vi "Control Bank Relays.vi"(8 "error in (no error)":errorcluster, 10 "bank params":T1, 11 "Refnum in":T4) -> (0 "error out":errorcluster)   [LabVIEW 2017, in "NI 272x Resistive Simulation Custom Device Engine.lvlib"]
uses:
  NI 272x Resistive Simulation Custom Device Engine.lvlib
  <instrlib>/ni272xReferenceVIs/ni272xReferenceVIs.llb/ni272x Reference.ctl
  bank params.ctl
  <vilib>/NI/NIVS Inline Async API/_Data Access Engine/Data Access Engine/Types/Read.DVR.ctl
  <vilib>/NI/NIVS Inline Async API/_Data Access Engine/Access Type Classes/Read/Read.lvclass
  Controls/Compiled Connect Channel.ctl
  <vilib>/NI/NIVS Inline Async API/_Data Access Engine/Access Type Classes/Read/Read.lvclass/Read.ctl
  <vilib>/NI/NIVS Inline Async API/_Data Access Engine/Data Access Engine/Methods/Read.Data.Detect.vi
  <vilib>/NI/NIVS Inline Async API/_Data Access Engine/Access Type Classes/Read/Read.ProcessData.Detect.vi
  <vilib>/NI/NIVS Inline Async API/_Data Access Engine/Data Access Engine/Data Access Engine.lvclass
  NI 272x Resistive Simulation Custom Device Shared.lvlib
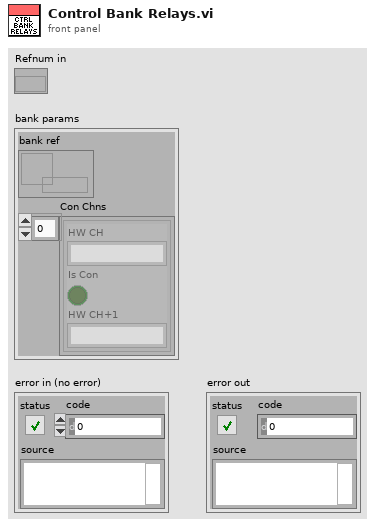
[diagram p1: front panel]
types:
  T1 = typedef "NI 272x Resistive Simulation Custom Device Engine.lvlib/bank params.ctl" = cluster{"bank ref":T2, "Con Chns":T3[]}
  T2 = typedef "Data Access Engine.lvlib/Data Access Engine.lvclass/Read.DVR.ctl" = refnum<data-value>
  T3 = typedef "NI 272x Resistive Simulation Custom Device Shared.lvlib/Compiled Connect Channel.ctl" = cluster{"HW CH":string, "Is Con":bool, "HW CH+1":string}
  T4 = typedef "ni272x Reference.ctl" = refnum<k20>
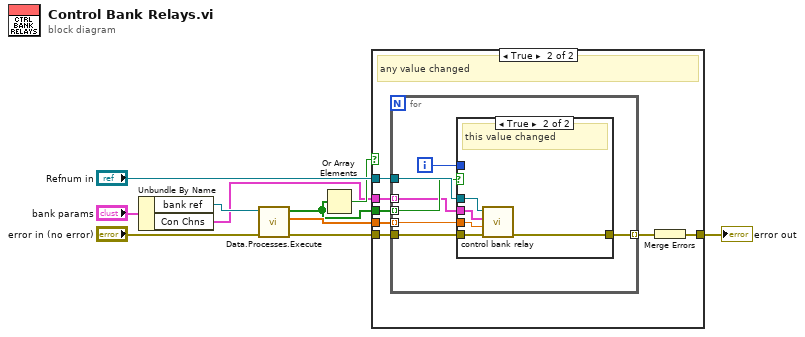
[diagram p0: block diagram]
diagram:
  n1 = Unbundle By Name("bank params") -> ("bank ref"=w2:T2, "Con Chns"=w1:T3[])
  n2 = call-poly <vilib>:"Data.Processes.Execute.vi"("error in (no error)"="error in (no error)", "Ref"=w2) -> ("error out"=w6:errorcluster, "Values"=w7:dbl[], "Detect?"=w5:bool[])  [unwired: 6 in, 1 out]
  n3 = Or Array Elements(Boolean array=w5) -> (logical OR=w4:bool)
  n4 = case shown="True" w4 {
    tunnel: [w11 w13] -> w10
    tunnel: w7 -> [_ w18]
    tunnel: "Refnum in" -> [_ w17]
    tunnel: w1 -> [_ w16]
    tunnel: w6 -> [w11 w14]
    tunnel: w5 -> [_ w12]
    frame False {
      # "no value change"
    }
    frame True {
      # "any value changed"
      n5 = for {
        tunnel: w12 -> [w24] mode=indexing
        tunnel: w18 -> [w22] mode=indexing
        tunnel: w17 -> [w25]
        tunnel: w16 -> [w23] mode=indexing
        tunnel: [w21] -> w15 mode=indexing
        tunnel: w14 -> [w20]
        i -> [w19]
        n6 = case shown="True" w24 {
          tunnel: w25 -> [_ w31]
          tunnel: w23 -> [_ w28]
          tunnel: w22 -> [_ w27]
          tunnel: [w26 w29] -> w21
          tunnel: w20 -> [w26 w30]
          tunnel: w19 -> [_ _]
          frame False {
            # "this value did not change"
          }
          frame True {
            # "this value changed"
            n7 = call "control bank relay.vi"("error in (no error)"=w30, "Channel Data Reference"=w27, "Connect Chn"=w28, "Refnum in"=w31) -> ("error out"=w29:errorcluster)  [unwired: 7 in]
          }
        }
      }
      n8 = Merge Errors(w15) -> (w13:errorcluster)
    }
  }
  "error out" <- w10
